vi "RichToFlatni_measurementlink_pinmap_v1_QueryRelaysRequest.vi"(5 "OutputClusterType":T1, 11 "InputCluster":T2) -> (3 "OutputCluster":T1)   [LabVIEW 2020, in "MeasurementLink Pin Map Client.lvlib"]
uses:
  MeasurementLink Pin Map Client.lvlib
  ni_measurementlink_pinmap_v1_QueryRelaysRequest.ctl
  ni_measurementlink_pinmap_v1_QueryRelaysRequest_Flat.ctl
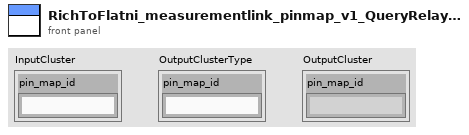
[diagram p1: front panel]
types:
  T1 = typedef "MeasurementLink Pin Map Client.lvlib/ni_measurementlink_pinmap_v1_QueryRelaysRequest_Flat.ctl" = cluster{"pin_map_id":string}
  T2 = typedef "MeasurementLink Pin Map Client.lvlib/ni_measurementlink_pinmap_v1_QueryRelaysRequest.ctl" = cluster{"pin_map_id":string}
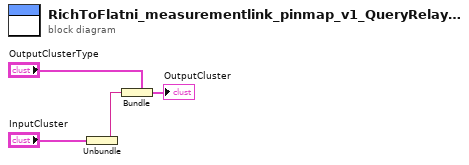
[diagram p0: block diagram]
diagram:
  n1 = Unbundle "Unbundle"("InputCluster") -> ("pin_map_id"=w1:string)
  n2 = Bundle "Bundle"(cluster="OutputClusterType", "pin_map_id"=w1) -> (→"OutputCluster":T1)
